vi "ZNA67_OneTrace_RS.vi"(5 "ZNA_Parameters":T2={"SweepPoints"=0, "StartFreq_GHz"=0.0, "StopFreq_GHz"=0.0, "S_Parameter"=0, "Marker_no."=1, "Marker_Freq(GHz)"=0.0}, 7 "ZNA_Func.":T3, 8 "error in":errorcluster, 11 "VISA IN":refnum<visa-resource-name>="TCPIP0::192.168.119.45::inst0::INSTR") -> (0 "error out":errorcluster, 1 "queryMarker":cluster{"gain":dbl, "phase":dbl} {"phase" format="%#.3f"; "gain" format="%#.3f"}, 2 "*OPC?":bool, 3 "Data":T1)   [LabVIEW 2023, in "R_S.lvlib"]
uses:
  R_S.lvlib
  CTL/RS_ZNA.ctl
panel:
  out "Duration(ms)":u32
  out "IDN":string
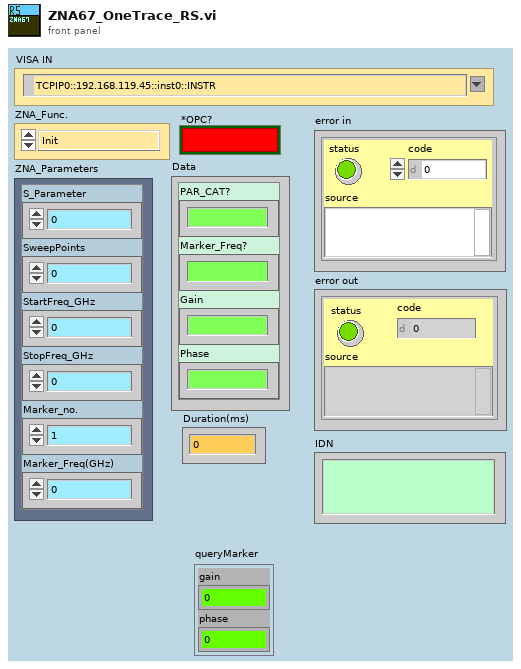
[diagram p1: front panel]
types:
  T1 = cluster{"PAR_CAT?":string, "Marker_Freq?":string, "Gain":string, "Phase":string}
  T2 = cluster{"SweepPoints":i32, "StartFreq_GHz":dbl, "StopFreq_GHz":dbl, "S_Parameter":i32, "Marker_no.":i32, "Marker_Freq(GHz)":dbl}
  T3 = typedef "RS_ZNA.ctl" = enum16{"Init", "Close", "set_SweepPoint", "set_MeasFormat", "set_FreqStartStop", "set_MeasPAR_S", "set_MarkerON", "set_MarkerOFF", "set_MarkerFreq", "set_MarkerFormat", "set_TriggerSingle", "query_GainPhase"}
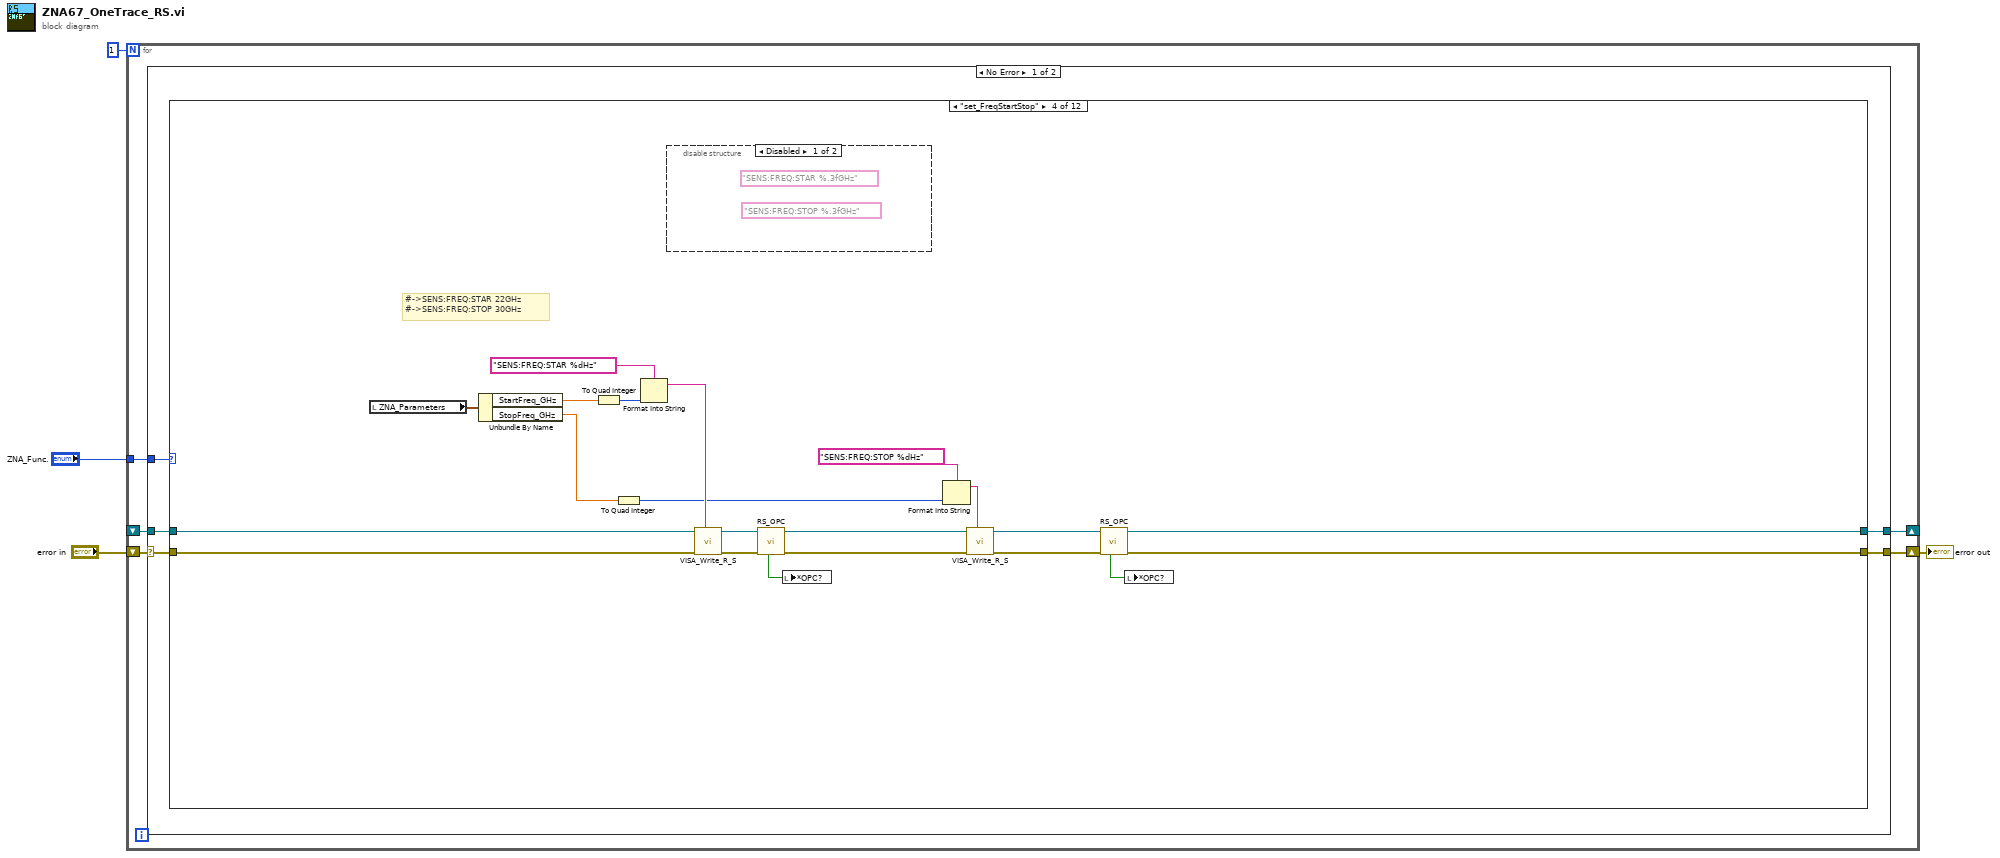
[diagram p0: block diagram]
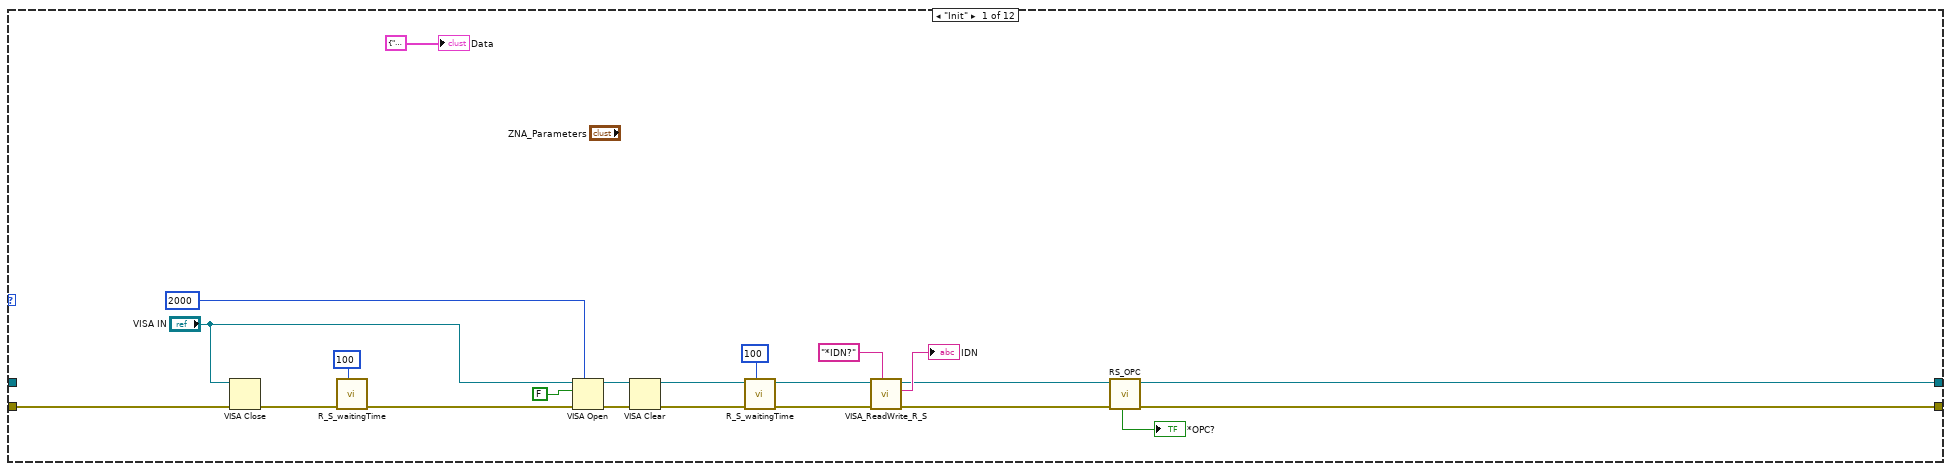
[diagram p2: hidden frame]
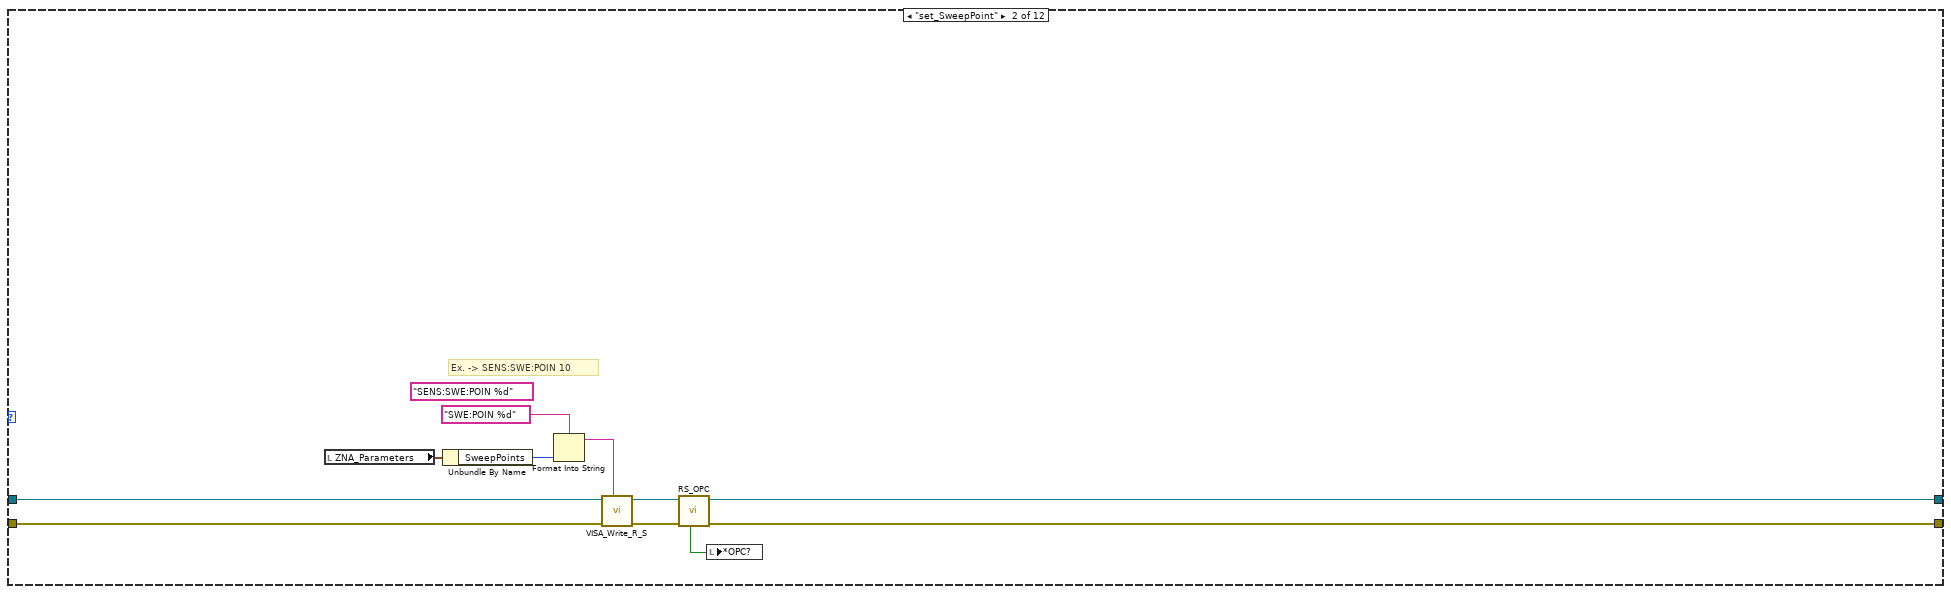
[diagram p3: hidden frame]
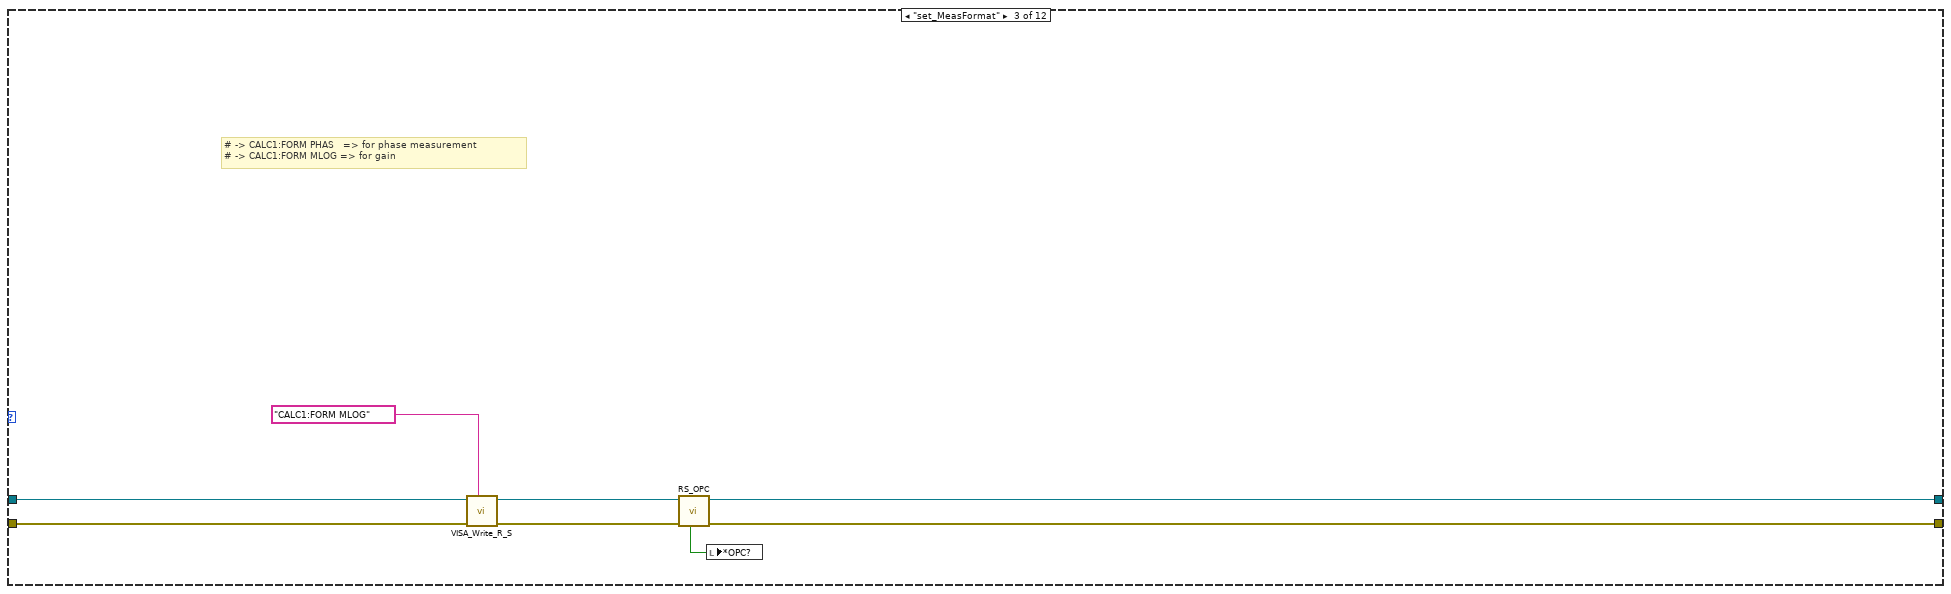
[diagram p4: hidden frame]
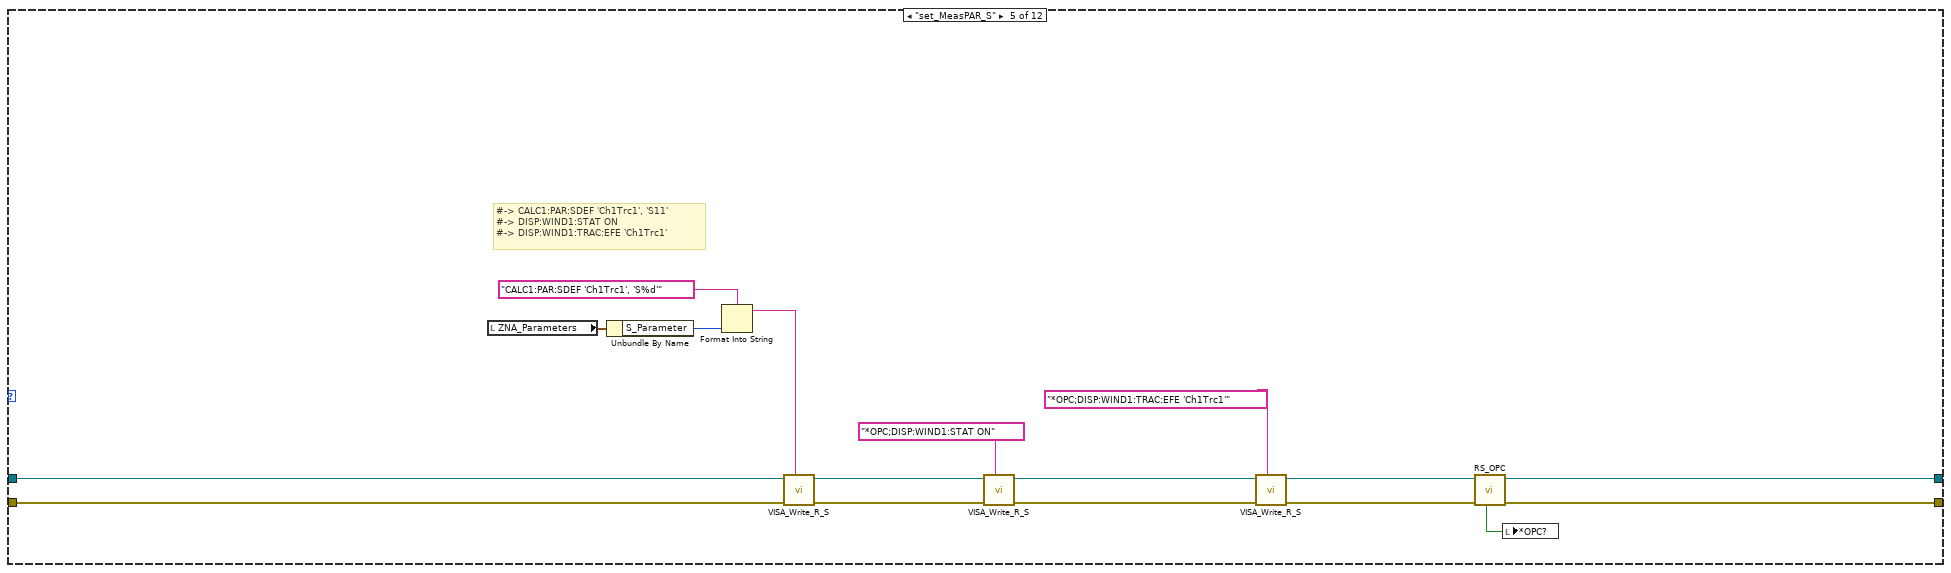
[diagram p6: hidden frame]
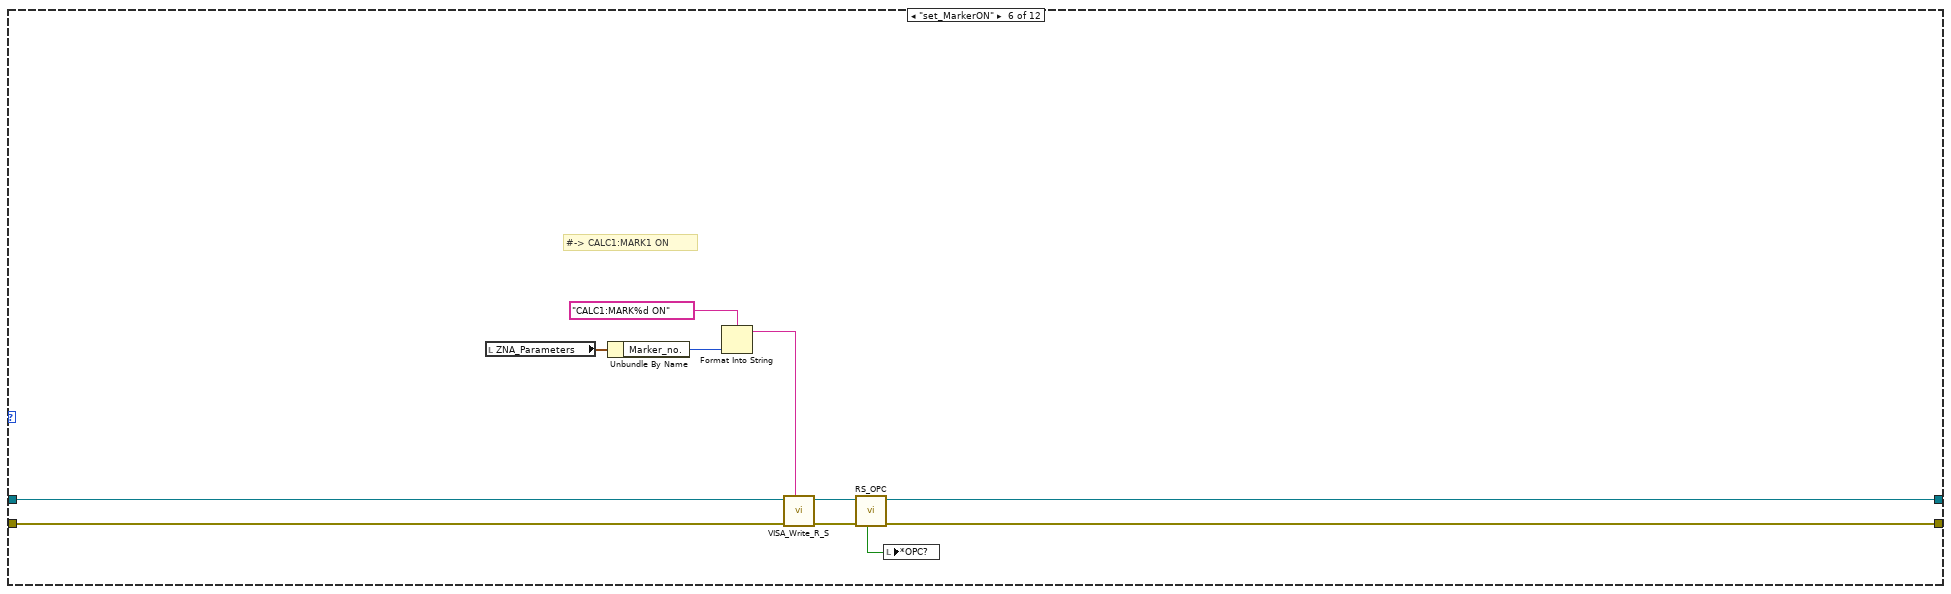
[diagram p7: hidden frame]
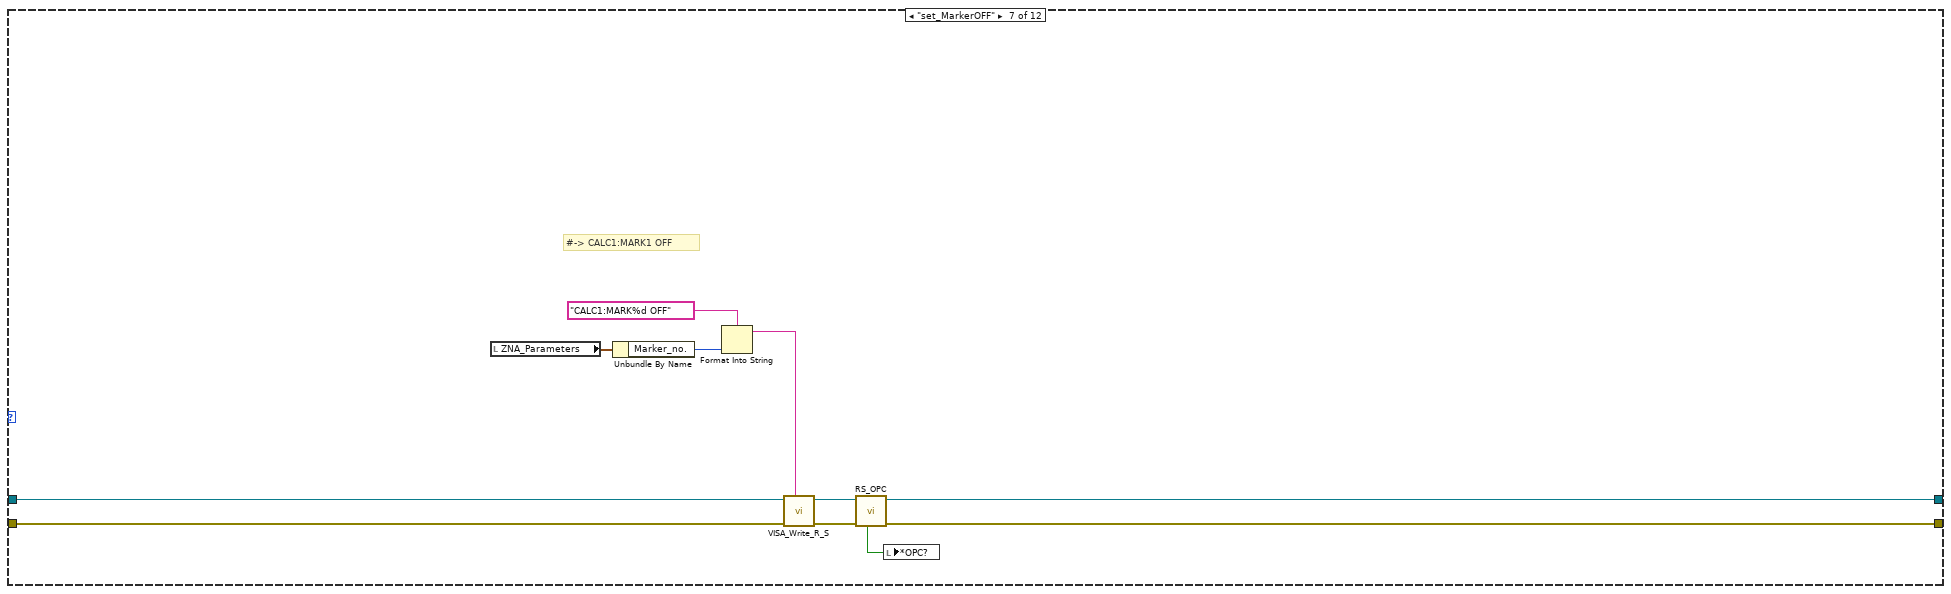
[diagram p8: hidden frame]
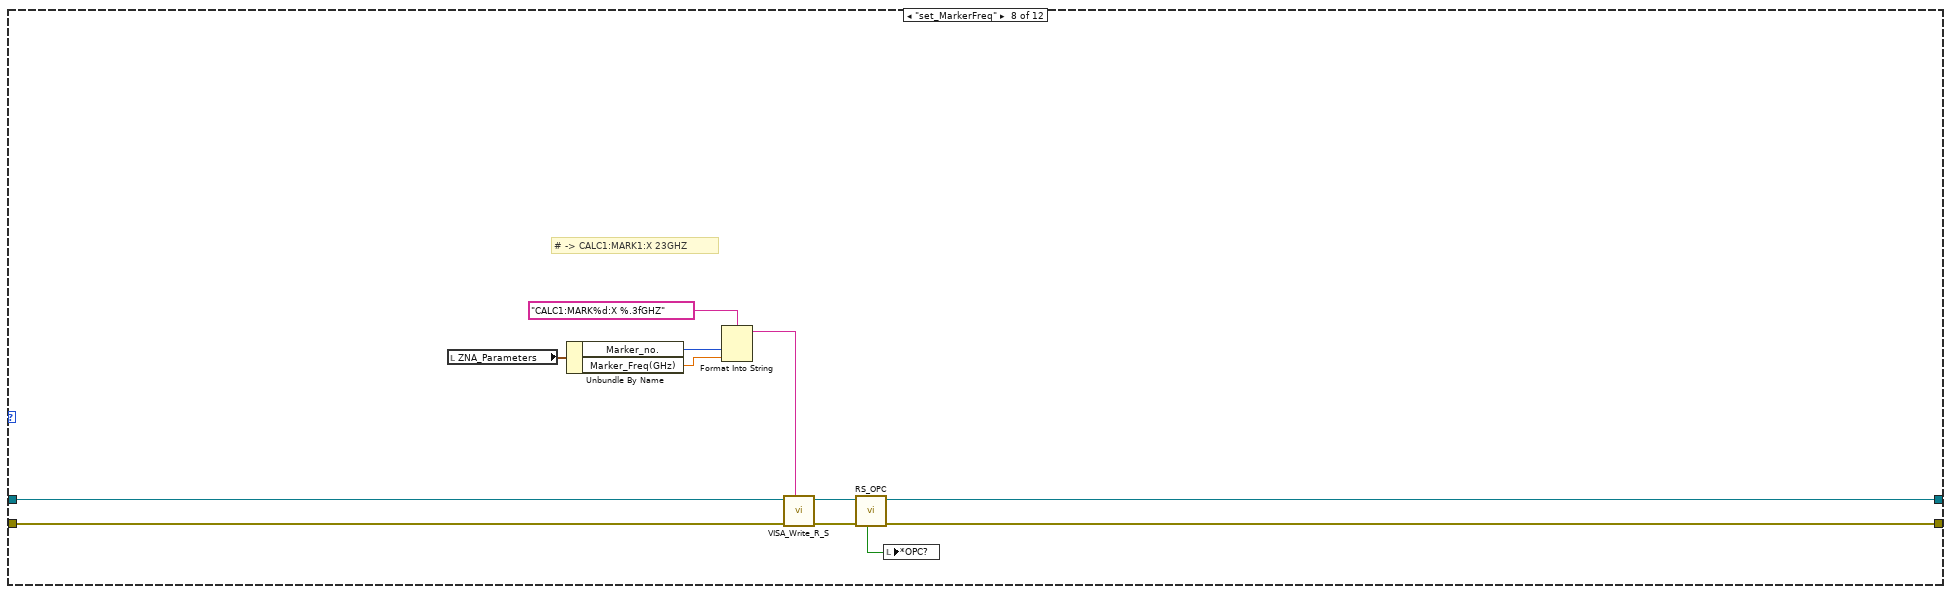
[diagram p9: hidden frame]
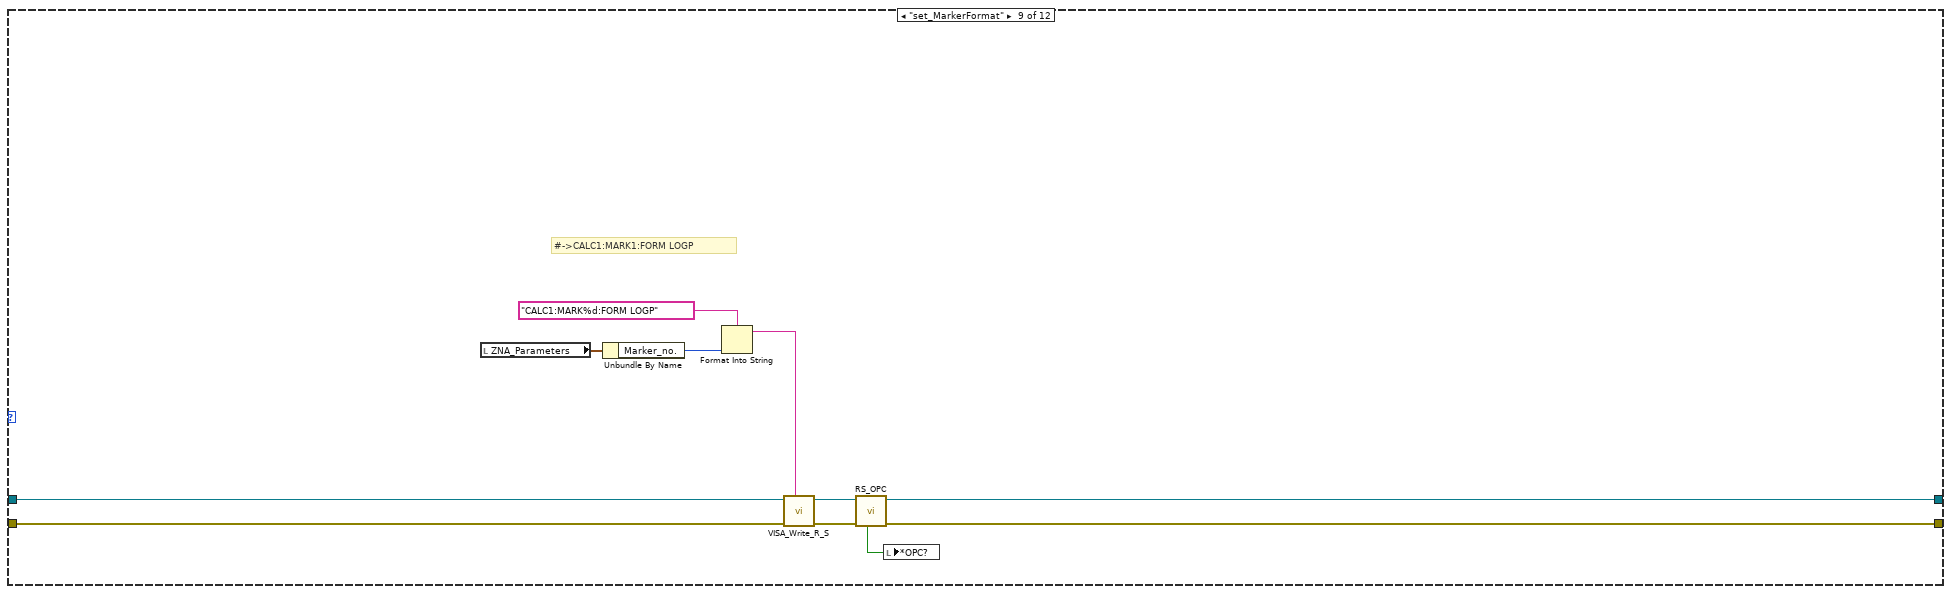
[diagram p10: hidden frame]
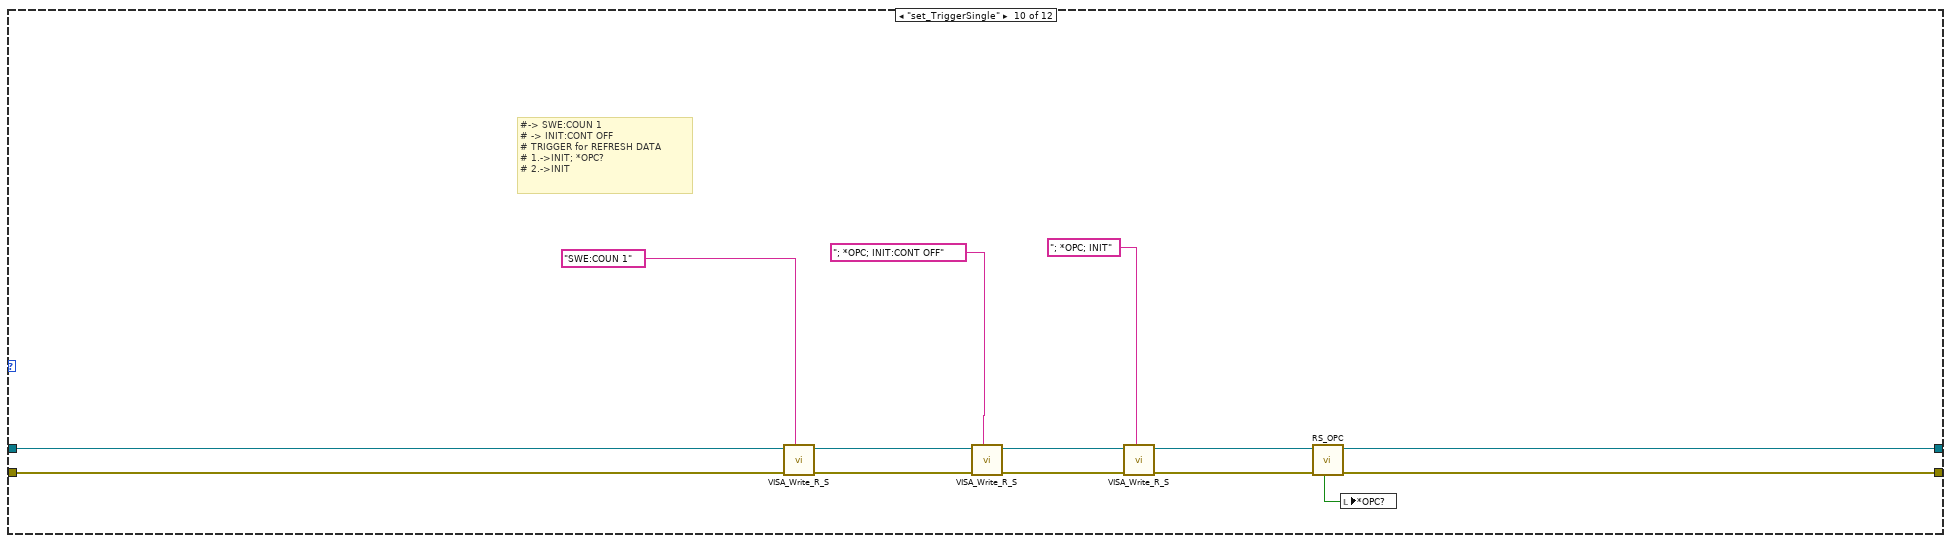
[diagram p11: hidden frame]
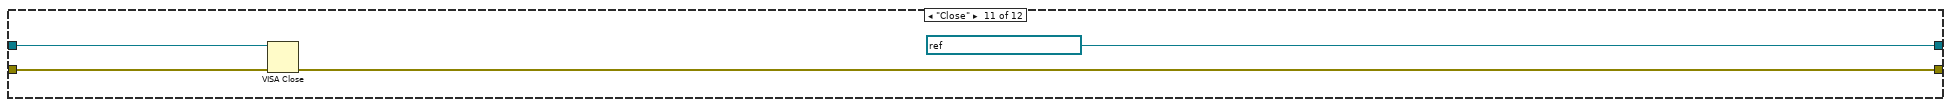
[diagram p12: hidden frame]
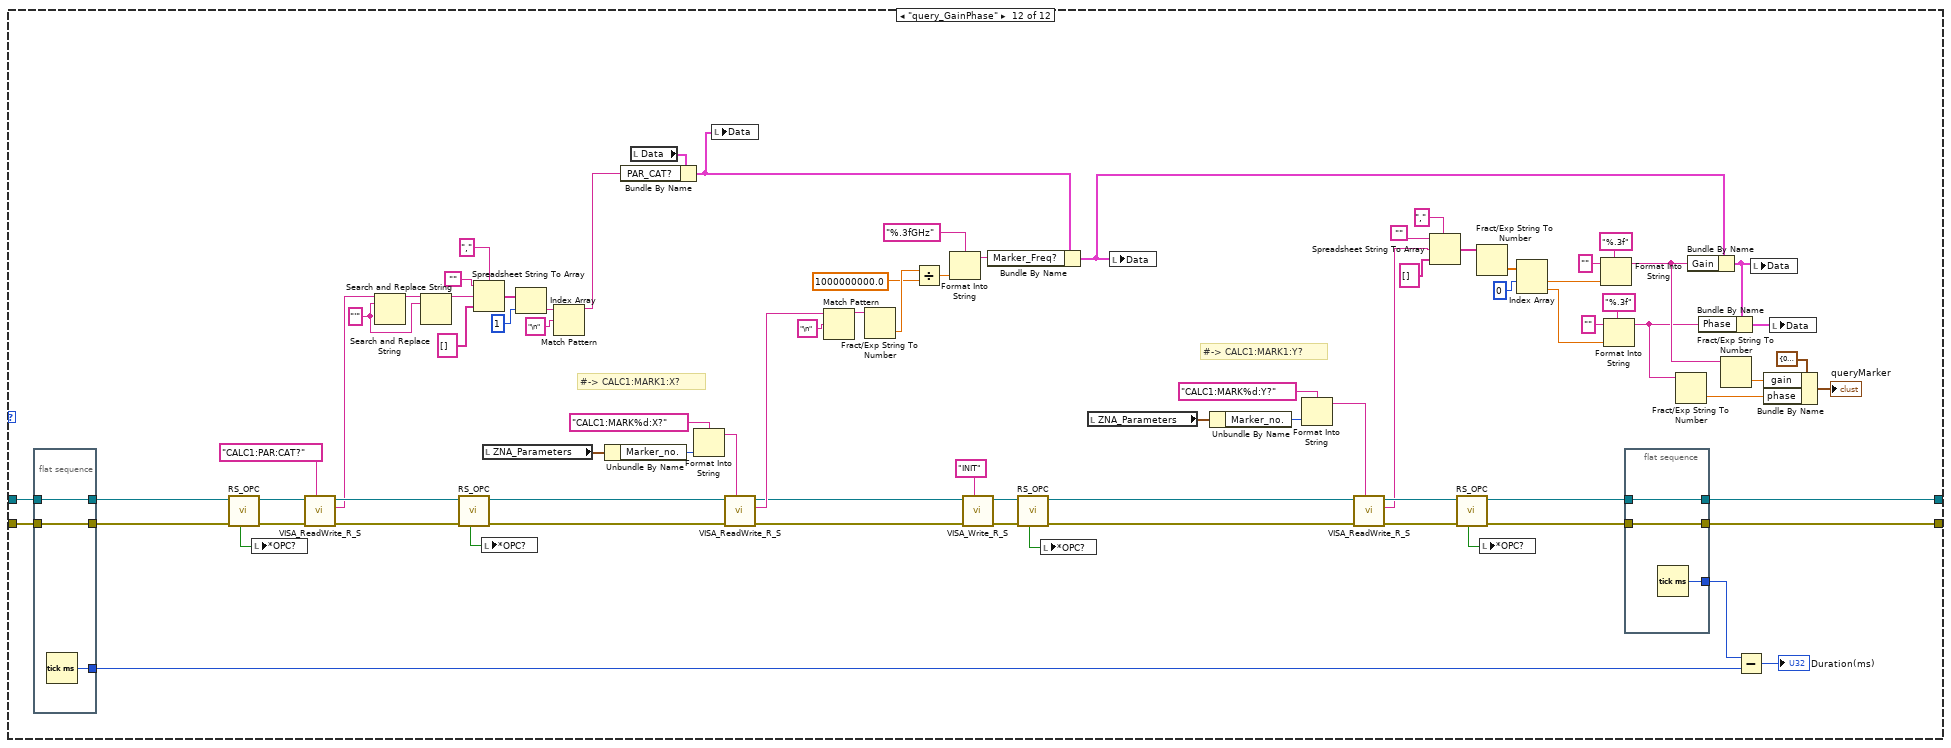
[diagram p13: hidden frame]
diagram:
  n1 = for {
    N: 1 -> [_]
    tunnel: "ZNA_Func." -> [w7]
    shift-right: [w8] -> w3
    shift-left: "error in" -> [w9]
    shift-right: [w5] -> _
    shift-left: _ -> [w6]
    n2 = case shown="No Error" w9 {
      selector: w9 -> [w13 w246]
      tunnel: [w12 w246] -> w8
      tunnel: w7 -> [w14 _]
      tunnel: w6 -> [w11 w245]
      tunnel: [w10 w245] -> w5
      frame No Error {
        n3 = case shown="\"set_FreqStartStop\"" w14 {
          tunnel: [w17 w39 w49 w61 w89 w98 w109 w121 w132 w148 w153 w170] -> w12
          tunnel: w13 -> [w28 w46 w54 w75 w92 w103 w114 w126 w137 w151 w155 w174]
          tunnel: w11 -> [_ w45 w53 w74 w91 w102 w113 w125 w136 w150 w154 w173]
          tunnel: [w18 w40 w50 w60 w90 w99 w110 w122 w133 w149 refnum<visa-resource-name> refnum ("VISA out") w169] -> w10
          frame "Init" {
            n4 = VISA Close(VISA resource name="VISA IN", error in (no error)=w28) -> (error out=w26:errorcluster)
            n5 = call "R_S_waitingTime.vi"("Waiting Time(ms)"=u32 100, "error in"=w26) -> ("error out"=w25:errorcluster)  [unwired: 9 in]
            n6 = VISA Open(timeout (0)=u32 2000 ("VISA Open timeout (0)"), duplicate session (F)=FALSE, error in (no error)=w25, VISA resource name="VISA IN") -> (VISA resource name=w32:refnum<visa-resource-name>, error out=w33:errorcluster)  [unwired: 1 in]
            n7 = VISA Clear(VISA resource name=w32, error in (no error)=w33) -> (VISA resource name out=w31:refnum<visa-resource-name>, error out=w22:errorcluster)
            n8 = call "R_S_waitingTime.vi"("Waiting Time(ms)"=u32 100, "error in"=w22) -> ("error out"=w21:errorcluster)  [unwired: 9 in]
            n9 = call "VISA_ReadWrite_R_S.vi"("VISA_CMD"="*IDN?", "error in"=w21, "VISA in"=w31) -> ("error out"=w20:errorcluster, "Response"=→"IDN":string, "VISA out"=w19:refnum<visa-resource-name>)  [unwired: 6 in]
            n10 = call "RS_OPC"("error in"=w20, "VISA in"=w19) -> ("error out"=w17:errorcluster, "VISA out"=w18:refnum<visa-resource-name>, "*OPC?"=→"*OPC?":bool)  [unwired: 6 in, 1 out]
            "Data" <- T1 {"PAR_CAT?"="", "Marker_Freq?"="", "Gain"="", "Phase"=""} ("Data")
          }
          frame "set_SweepPoint" {
            (unwired) "SENS:SWE:POIN %d" ("VISA CMD")
            # "Ex. -> SENS:SWE:POIN 10"
            n11 = local read "ZNA_Parameters"() -> (w37:T2)
            n12 = Unbundle By Name(w37) -> ("SweepPoints"=w36:i32)
            n13 = Format Into String(format string="SWE:POIN %d" ("VISA CMD"), w36) -> (resulting string=w43:string)  [unwired: 2 in, 1 out]
            n14 = call "VISA_Write_R_S.vi"("VISA CMD"=w43, "error in"=w46, "VISA in"=w45) -> ("error out"=w42:errorcluster, "VISA out"=w41:refnum<visa-resource-name>)  [unwired: 7 in]
            n15 = call "RS_OPC"("error in"=w42, "VISA in"=w41) -> ("error out"=w39:errorcluster, "VISA out"=w40:refnum<visa-resource-name>, "*OPC?"=w38:bool)  [unwired: 6 in, 1 out]
            n16 = local write "*OPC?"(w38) -> ()
          }
          frame "set_MeasFormat" {
            # "# -> CALC1:FORM PHAS   => for phase measurement\n# -> CALC1:FORM MLOG => for gain"
            n17 = call "VISA_Write_R_S.vi"("VISA CMD"="CALC1:FORM MLOG", "error in"=w54, "VISA in"=w53) -> ("error out"=w52:errorcluster, "VISA out"=w51:refnum<visa-resource-name>)  [unwired: 7 in]
            n18 = call "RS_OPC"("error in"=w52, "VISA in"=w51) -> ("error out"=w49:errorcluster, "VISA out"=w50:refnum<visa-resource-name>, "*OPC?"=w48:bool)  [unwired: 6 in, 1 out]
            n19 = local write "*OPC?"(w48) -> ()
          }
          frame "set_FreqStartStop" {
            # "#->SENS:FREQ:STAR 22GHz\n#->SENS:FREQ:STOP 30GHz"
            n20 = local read "ZNA_Parameters"() -> (w59:T2)
            n21 = Unbundle By Name(w59) -> ("StartFreq_GHz"=w57:dbl, "StopFreq_GHz"=w58:dbl)
            n22 = To Quad Integer(1:w57) -> (0:w56:i64)
            n23 = To Quad Integer(1:w58) -> (0:w55:i64)
            n24 = Format Into String(format string="SENS:FREQ:STAR %dHz" ("VISA CMD"), w56) -> (resulting string=w70:string)  [unwired: 2 in, 1 out]
            n25 = disable-structure shown="Disabled" {
              frame Disabled {
                (unwired) "SENS:FREQ:STAR %.3fGHz" ("VISA CMD")
                (unwired) "SENS:FREQ:STOP %.3fGHz"
              }
              frame Enabled {
              }
            }
            n26 = call "VISA_Write_R_S.vi"("VISA CMD"=w70, "error in"=w75, "VISA in"=w74) -> ("error out"=w73:errorcluster, "VISA out"=w72:refnum<visa-resource-name>)  [unwired: 7 in]
            n27 = call "RS_OPC"("error in"=w73, "VISA in"=w72) -> ("error out"=w68:errorcluster, "VISA out"=w67:refnum<visa-resource-name>, "*OPC?"=w71:bool)  [unwired: 6 in, 1 out]
            n28 = local write "*OPC?"(w71) -> ()
            n29 = Format Into String(format string="SENS:FREQ:STOP %dHz", w55) -> (resulting string=w66:string)  [unwired: 2 in, 1 out]
            n30 = call "VISA_Write_R_S.vi"("VISA CMD"=w66, "error in"=w68, "VISA in"=w67) -> ("error out"=w62:errorcluster, "VISA out"=w63:refnum<visa-resource-name>)  [unwired: 7 in]
            n31 = call "RS_OPC"("error in"=w62, "VISA in"=w63) -> ("error out"=w61:errorcluster, "VISA out"=w60:refnum<visa-resource-name>, "*OPC?"=w64:bool)  [unwired: 6 in, 1 out]
            n32 = local write "*OPC?"(w64) -> ()
          }
          frame "set_MeasPAR_S" {
            # "#-> CALC1:PAR:SDEF 'Ch1Trc1', 'S11'\n#-> DISP:WIND1:STAT ON\n#-> DISP:WIND1:TRAC:EFE 'Ch1Trc1'"
            n33 = local read "ZNA_Parameters"() -> (w77:T2)
            n34 = Unbundle By Name(w77) -> ("S_Parameter"=w76:i32)
            n35 = Format Into String(format string="CALC1:PAR:SDEF 'Ch1Trc1', 'S%d'" ("VISA CMD"), w76) -> (resulting string=w87:string)  [unwired: 2 in, 1 out]
            n36 = call "VISA_Write_R_S.vi"("VISA CMD"=w87, "error in"=w92, "VISA in"=w91) -> ("error out"=w85:errorcluster, "VISA out"=w84:refnum<visa-resource-name>)  [unwired: 7 in]
            n37 = call "VISA_Write_R_S.vi"("VISA CMD"="*OPC;DISP:WIND1:STAT ON", "error in"=w85, "VISA in"=w84) -> ("error out"=w82:errorcluster, "VISA out"=w80:refnum<visa-resource-name>)  [unwired: 7 in]
            n38 = call "VISA_Write_R_S.vi"("VISA CMD"="*OPC;DISP:WIND1:TRAC:EFE 'Ch1Trc1'", "error in"=w82, "VISA in"=w80) -> ("error out"=w81:errorcluster, "VISA out"=w79:refnum<visa-resource-name>)  [unwired: 7 in]
            n39 = call "RS_OPC"("error in"=w81, "VISA in"=w79) -> ("error out"=w89:errorcluster, "VISA out"=w90:refnum<visa-resource-name>, "*OPC?"=w88:bool)  [unwired: 6 in, 1 out]
            n40 = local write "*OPC?"(w88) -> ()
          }
          frame "set_MarkerON" {
            # "#-> CALC1:MARK1 ON"
            n41 = local read "ZNA_Parameters"() -> (w94:T2)
            n42 = Unbundle By Name(w94) -> ("Marker_no."=w93:i32)
            n43 = Format Into String(format string="CALC1:MARK%d ON" ("VISA CMD"), w93) -> (resulting string=w96:string)  [unwired: 2 in, 1 out]
            n44 = call "VISA_Write_R_S.vi"("VISA CMD"=w96, "error in"=w103, "VISA in"=w102) -> ("error out"=w101:errorcluster, "VISA out"=w100:refnum<visa-resource-name>)  [unwired: 7 in]
            n45 = call "RS_OPC"("error in"=w101, "VISA in"=w100) -> ("error out"=w98:errorcluster, "VISA out"=w99:refnum<visa-resource-name>, "*OPC?"=w97:bool)  [unwired: 6 in, 1 out]
            n46 = local write "*OPC?"(w97) -> ()
          }
          frame "set_MarkerOFF" {
            # "#-> CALC1:MARK1 OFF"
            n47 = local read "ZNA_Parameters"() -> (w105:T2)
            n48 = Unbundle By Name(w105) -> ("Marker_no."=w104:i32)
            n49 = Format Into String(format string="CALC1:MARK%d OFF" ("VISA CMD"), w104) -> (resulting string=w107:string)  [unwired: 2 in, 1 out]
            n50 = call "VISA_Write_R_S.vi"("VISA CMD"=w107, "error in"=w114, "VISA in"=w113) -> ("error out"=w112:errorcluster, "VISA out"=w111:refnum<visa-resource-name>)  [unwired: 7 in]
            n51 = call "RS_OPC"("error in"=w112, "VISA in"=w111) -> ("error out"=w109:errorcluster, "VISA out"=w110:refnum<visa-resource-name>, "*OPC?"=w108:bool)  [unwired: 6 in, 1 out]
            n52 = local write "*OPC?"(w108) -> ()
          }
          frame "set_MarkerFreq" {
            # "# -> CALC1:MARK1:X 23GHZ"
            n53 = local read "ZNA_Parameters"() -> (w117:T2)
            n54 = Unbundle By Name(w117) -> ("Marker_no."=w116:i32, "Marker_Freq(GHz)"=w115:dbl)
            n55 = Format Into String(format string="CALC1:MARK%d:X %.3fGHZ" ("VISA CMD"), w116, w115) -> (resulting string=w119:string)  [unwired: 2 in, 1 out]
            n56 = call "VISA_Write_R_S.vi"("VISA CMD"=w119, "error in"=w126, "VISA in"=w125) -> ("error out"=w124:errorcluster, "VISA out"=w123:refnum<visa-resource-name>)  [unwired: 7 in]
            n57 = call "RS_OPC"("error in"=w124, "VISA in"=w123) -> ("error out"=w121:errorcluster, "VISA out"=w122:refnum<visa-resource-name>, "*OPC?"=w120:bool)  [unwired: 6 in, 1 out]
            n58 = local write "*OPC?"(w120) -> ()
          }
          frame "set_MarkerFormat" {
            # "#->CALC1:MARK1:FORM LOGP"
            n59 = local read "ZNA_Parameters"() -> (w128:T2)
            n60 = Unbundle By Name(w128) -> ("Marker_no."=w127:i32)
            n61 = Format Into String(format string="CALC1:MARK%d:FORM LOGP" ("VISA CMD"), w127) -> (resulting string=w130:string)  [unwired: 2 in, 1 out]
            n62 = call "VISA_Write_R_S.vi"("VISA CMD"=w130, "error in"=w137, "VISA in"=w136) -> ("error out"=w135:errorcluster, "VISA out"=w134:refnum<visa-resource-name>)  [unwired: 7 in]
            n63 = call "RS_OPC"("error in"=w135, "VISA in"=w134) -> ("error out"=w132:errorcluster, "VISA out"=w133:refnum<visa-resource-name>, "*OPC?"=w131:bool)  [unwired: 6 in, 1 out]
            n64 = local write "*OPC?"(w131) -> ()
          }
          frame "set_TriggerSingle" {
            # "#-> SWE:COUN 1\n# -> INIT:CONT OFF\n# TRIGGER for REFRESH DATA\n# 1.->INIT; *OPC?\n# 2.->INIT"
            n65 = call "VISA_Write_R_S.vi"("VISA CMD"="SWE:COUN 1", "error in"=w151, "VISA in"=w150) -> ("error out"=w145:errorcluster, "VISA out"=w143:refnum<visa-resource-name>)  [unwired: 7 in]
            n66 = call "VISA_Write_R_S.vi"("VISA CMD"="; *OPC; INIT:CONT OFF", "error in"=w145, "VISA in"=w143) -> ("error out"=w146:errorcluster, "VISA out"=w144:refnum<visa-resource-name>)  [unwired: 7 in]
            n67 = call "VISA_Write_R_S.vi"("VISA CMD"="; *OPC; INIT", "error in"=w146, "VISA in"=w144) -> ("error out"=w141:errorcluster, "VISA out"=w142:refnum<visa-resource-name>)  [unwired: 7 in]
            n68 = call "RS_OPC"("error in"=w141, "VISA in"=w142) -> ("error out"=w148:errorcluster, "VISA out"=w149:refnum<visa-resource-name>, "*OPC?"=w147:bool)  [unwired: 6 in, 1 out]
            n69 = local write "*OPC?"(w147) -> ()
          }
          frame "Close" {
            n70 = VISA Close(VISA resource name=w154, error in (no error)=w155) -> (error out=w153:errorcluster)
          }
          frame "query_GainPhase" {
            w193 = "'" ("search string")
            # "#-> CALC1:MARK1:Y?"
            # "#-> CALC1:MARK1:X?"
            n71 = flat-sequence {
              tunnel: w174 -> [w244]
              tunnel: [w244] -> w164
              tunnel: w173 -> [w243]
              tunnel: [w243] -> w165
              tunnel: [w242] -> w167
              frame #0 {
                n72 = Tick Count (ms)() -> (millisecond timer value=w242:u32)
              }
            }
            n73 = call "RS_OPC"("error in"=w164, "VISA in"=w165) -> ("error out"=w237:errorcluster, "VISA out"=w236:refnum<visa-resource-name>, "*OPC?"=w238:bool)  [unwired: 6 in, 1 out]
            n74 = local write "*OPC?"(w238) -> ()
            n75 = call "VISA_ReadWrite_R_S.vi"("VISA_CMD"="CALC1:PAR:CAT?", "error in"=w237, "VISA in"=w236) -> ("error out"=w228:errorcluster, "Response"=w191:string, "VISA out"=w227:refnum<visa-resource-name>)  [unwired: 6 in]
            n76 = Search and Replace String(input string=w191, search string=w193) -> (result string=w194:string)  [unwired: 6 in, 3 out]
            n77 = Search and Replace String(input string=w194, search string=w193) -> (result string=w190:string)  [unwired: 6 in, 3 out]
            n78 = call "RS_OPC"("error in"=w228, "VISA in"=w227) -> ("error out"=w226:errorcluster, "VISA out"=w225:refnum<visa-resource-name>, "*OPC?"=w229:bool)  [unwired: 6 in, 1 out]
            n79 = Spreadsheet String To Array(delimiter (Tab)="," ("spreadsheet string"), format string="", spreadsheet string=w190, array type (2D Dbl)=string[] []) -> (array=w232:string[])
            n80 = local write "*OPC?"(w229) -> ()
            n81 = local read "ZNA_Parameters"() -> (w185:T2)
            n82 = Index Array(array=w232, index=1) -> (element=w230:string)
            n83 = Match Pattern(string=w230, regular expression="\n") -> (before substring=w181:string)  [unwired: 1 in, 3 out]
            n84 = Unbundle By Name(w185) -> ("Marker_no."=w184:i32)
            n85 = local read "Data"() -> (w178:T1)
            n86 = Bundle By Name(cluster=w178, "PAR_CAT?"=w181) -> (w177:T1)
            n87 = Format Into String(format string="CALC1:MARK%d:X?" ("VISA CMD"), w184) -> (resulting string=w223:string)  [unwired: 2 in, 1 out]
            n88 = local write "Data"(w177) -> ()
            n89 = call "VISA_ReadWrite_R_S.vi"("VISA_CMD"=w223, "error in"=w226, "VISA in"=w225) -> ("error out"=w215:errorcluster, "Response"=w221:string, "VISA out"=w214:refnum<visa-resource-name>)  [unwired: 6 in]
            n90 = Match Pattern(string=w221, regular expression="\n") -> (before substring=w220:string)  [unwired: 1 in, 3 out]
            n91 = Fract/Exp String To Number(string=w220) -> (number=w218:dbl)  [unwired: 3 in, 1 out]
            n92 = Divide(x=w218, y=1000000000.0) -> (x/y=w216:dbl)
            n93 = Format Into String(format string="%.3fGHz" ("VISA CMD"), w216) -> (resulting string=w180:string)  [unwired: 2 in, 1 out]
            n94 = call "VISA_Write_R_S.vi"("VISA CMD"="INIT", "error in"=w215, "VISA in"=w214) -> ("error out"=w212:errorcluster, "VISA out"=w211:refnum<visa-resource-name>)  [unwired: 7 in]
            n95 = Bundle By Name(cluster=w177, "Marker_Freq?"=w180) -> (w176:T1)
            n96 = call "RS_OPC"("error in"=w212, "VISA in"=w211) -> ("error out"=w208:errorcluster, "VISA out"=w207:refnum<visa-resource-name>, "*OPC?"=w210:bool)  [unwired: 6 in, 1 out]
            n97 = local write "*OPC?"(w210) -> ()
            n98 = local read "ZNA_Parameters"() -> (w183:T2)
            n99 = local write "Data"(w176) -> ()
            n100 = Unbundle By Name(w183) -> ("Marker_no."=w182:i32)
            n101 = Format Into String(format string="CALC1:MARK%d:Y?" ("VISA CMD"), w182) -> (resulting string=w206:string)  [unwired: 2 in, 1 out]
            n102 = call "VISA_ReadWrite_R_S.vi"("VISA_CMD"=w206, "error in"=w208, "VISA in"=w207) -> ("error out"=w196:errorcluster, "Response"=w187:string, "VISA out"=w195:refnum<visa-resource-name>)  [unwired: 6 in]
            n103 = Spreadsheet String To Array(delimiter (Tab)="," ("spreadsheet string"), format string="", spreadsheet string=w187, array type (2D Dbl)=string[] []) -> (array=w203:string[])
            n104 = call "RS_OPC"("error in"=w196, "VISA in"=w195) -> ("error out"=w172:errorcluster, "VISA out"=w171:refnum<visa-resource-name>, "*OPC?"=w197:bool)  [unwired: 6 in, 1 out]
            n105 = Fract/Exp String To Number(string=w203) -> (number=w202:dbl[])  [unwired: 3 in, 1 out]
            n106 = local write "*OPC?"(w197) -> ()
            n107 = Index Array(array=w202, index #1=0 ("index")) -> (element #1=w161:dbl, element #2=w160:dbl)  [unwired: 1 in]
            n108 = Format Into String(format string="%.3f" ("VISA CMD"), initial string="", w161) -> (resulting string=w159:string)  [unwired: 1 in, 1 out]
            n109 = Format Into String(format string="%.3f" ("VISA CMD"), initial string="", w160) -> (resulting string=w157:string)  [unwired: 1 in, 1 out]
            n110 = flat-sequence {
              tunnel: w172 -> [w241]
              tunnel: [w241] -> w170
              tunnel: w171 -> [w240]
              tunnel: [w240] -> w169
              tunnel: [w239] -> w168
              frame #0 {
                n111 = Tick Count (ms)() -> (millisecond timer value=w239:u32)
              }
            }
            n112 = Fract/Exp String To Number(string=w157) -> (number=w156:dbl)  [unwired: 3 in, 1 out]
            n113 = Bundle By Name(cluster=w176, "Gain"=w159) -> (w175:T1)
            n114 = Bundle By Name(cluster=w175, "Phase"=w157) -> (w179:T1)
            n115 = Fract/Exp String To Number(string=w159) -> (number=w158:dbl)  [unwired: 3 in, 1 out]
            n116 = Subtract(x=w168, y=w167) -> (x-y=→"Duration(ms)":u32)
            n117 = local write "Data"(w175) -> ()
            n118 = Bundle By Name(cluster=cluster{"gain":dbl, "phase":dbl} {"gain"=0.0, "phase"=0.0} ("queryMarker 2"), "gain"=w158, "phase"=w156) -> (→"queryMarker":cluster{"gain":dbl, "phase":dbl})
            n119 = local write "Data"(w179) -> ()
          }
        }
      }
      frame Error {
      }
    }
  }
  "error out" <- w3
